vi "main.vi"() -> ()   [LabVIEW 2009, in "NavScreen.lvlib"]
uses:
  NavScreen.lvlib
  ItemIcon.ctl
  Classes/Link/Link.lvclass
  Classes/RingItem/RingItem.lvclass
panel:
  in  "stop":bool
  in  "Launch Project Wizard for Target":bool
  in  "Target Devices":u16(ring) items=["Real-Time Project"]
  in  "DNL_Column1Section3TopAlignment":bool caption="Find Examples..."
  in  "DNL_FileColumnLeftAlignment":string
  in  "DNL_ResourceColumnLeftAlignment":string
  in  "Ring 2-13":T1
  in  "Ring 2-14":T1
  in  "Ring 2-15":T1
  in  "Ring 2-16":T1
  in  "Ring 2-11":T1
  in  "Ring 2-10":T1
  in  "Ring 2-9":T1
  in  "Ring 2-8":T1
  in  "Ring 2-7":T1
  in  "Ring 2-6":T1
  in  "Ring 2-5":T1
  out "File":string="Column One"
  out "Resources":string="Column Two"
  in  "DNL_Link Button 25":bool caption="New To LabVIEW?"
  in  "DNL_Link Button 26":bool caption="Getting Started with LabVIEW"
  in  "DNL_Link Button 27":bool caption="LabVIEW Fundamentals"
  in  "DNL_Link Button 28":bool caption="Guide to LabVIEW Documentation"
  in  "DNL_Link Button 29":bool caption="LabVIEW Help"
  in  "DNL_Link Button 30":bool caption="Web Links"
  in  "DNL_Link Button 31":bool caption="Eyes on VIs (LabVIEW Blog)"
  in  "DNL_Link Button 32":bool caption="Darren's Weekly Nuggets"
  in  "DNL_Link Button 33":bool caption="LAVA"
  in  "DNL_Link Button 34":bool caption="LabVIEW Wiki"
  in  "DNL_Link Button 35":bool caption="More Web Resources"
  in  "DNL_Link Button 36":bool caption="Discussion Forums"
  in  "DNL_Link Button 37":bool caption="Training Courses"
  in  "DNL_Link Button 38":bool caption="LabVIEW Zone"
  in  "DNL_Link Button 39":bool caption="More Blogs"
  in  "DNL_Link Button 40":bool caption="NI Blog Listing"
  in  "DNL_Link Button 15":bool caption="Find Examples..."
  in  "DNL_Link Button 14":bool caption="Examples"
  in  "DNL_Link Button 13":bool caption="Browse..."
  in  "DNL_Link Button 12":bool caption="Untitled2.vi"
  in  "DNL_Link Button 11":bool caption="Targets"
  in  "DNL_Link Button 10":bool caption="Placeholder"
  in  "DNL_Link Button 9":bool caption="Placeholder"
  in  "DNL_Link Button 8":bool caption="Targets"
  in  "DNL_Link Button 7":bool caption="Browse..."
  in  "DNL_Link Button 6":bool caption="Section Header 2"
  in  "DNL_Link Button 5":bool caption="More..."
  in  "DNL_Link Button 4":bool caption="Placeholder"
  in  "DNL_Link Button 3":bool caption="Placeholder"
  in  "DNL_Link Button 2":bool caption="Real-Time Project"
  in  "DNL_Link Button 1":bool caption="Section Header"
  in  "DNL_Link Button 41":bool
  in  "DNL_Link Button 42":bool
  in  "DNL_Link Button 43":bool
  in  "DNL_Link Button 44":bool
  in  "DNL_Link Button 45":bool
  in  "DNL_Link Button 46":bool
  in  "DNL_Link Button 47":bool
  in  "DNL_Link Button 48":bool
  in  "DNL_Link Button 16":bool
  in  "DNL_Link Button 24":bool
  in  "DNL_Link Button 23":bool
  in  "DNL_Link Button 22":bool
  in  "DNL_Link Button 21":bool
  in  "DNL_Link Button 20":bool
  in  "DNL_Link Button 19":bool
  in  "DNL_Link Button 18":bool
  in  "DNL_Link Button 17":bool
  in  "Ring 2-4":T1
  in  "Ring 2-3":T1=1
  in  "Ring 2-2":T1=1
  in  "Ring 2":T1=8
  in  "Ring 2-12":T1
  out "Getting Started window":u16(ring)=2
  # "We size and scroll the panel programmatically during initialization. The background below is a picture ring.\n\nThe (off-screen) controls below define the left position of the two columns."
  # "This example demonstrates several aspects of LabVIEW object-oriented programming.\n\nIt is similar to the implementation of the LabVIEW Getting Started window.\n\nAn instance of a LabVIEW class handles each link on the dialog. Different classes handle different kinds of links (web URLs, help files, etc). All the classes inherit from Link.lvclass.\n\nThe private data of each class holds the information needed to perform the work of that class. For example, the Web.lvclass private data includes the URL to open.\n\nThe classes employ two kinds of dynamically dispatching member VIs. Some dynamic dispatching member VIs build upon the parent implementation of the VI, while others replace the parent implementation. The InitFromXML VIs extend the functionality of the parent classes by calling the parent implementation of the method and then doing additional work. The HandleItemActivation VIs override the parent class, substituting its work for whatever the parent class would have done in its absence.\n\nThe LinkItemFromXML.vi in Link.lvclass illustrates a \"factory\" design pattern.\n\nFinally, ProjectWizard.lvclass illustrates a helper class, allowing ProjectWizardClickableText.lvclass and RingItemProjectWizard.lvclass to share functionality without having a unique common ancestor class."
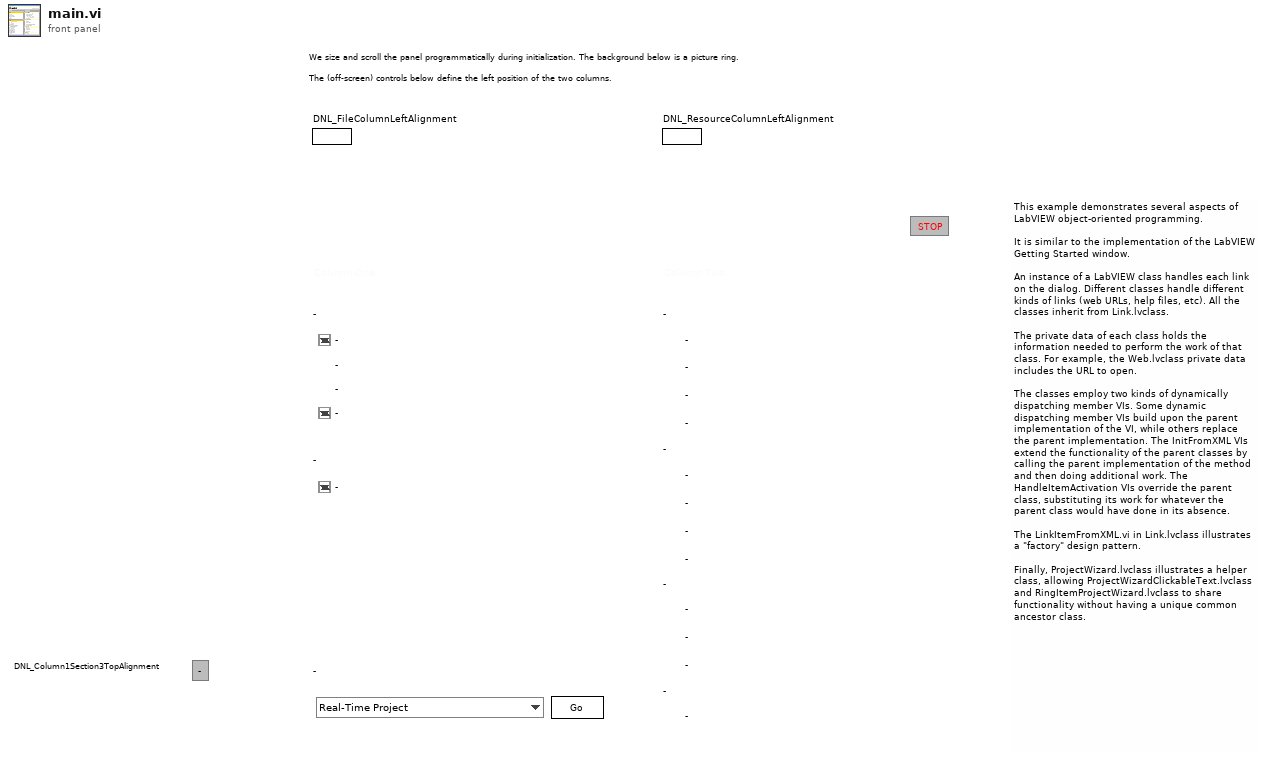
[diagram p1: front panel]
types:
  T1 = typedef "NavScreen.lvlib/ItemIcon.ctl" = u16
  T2 = cluster{refnum<class "ClickableText.lvclass">[]}[][]
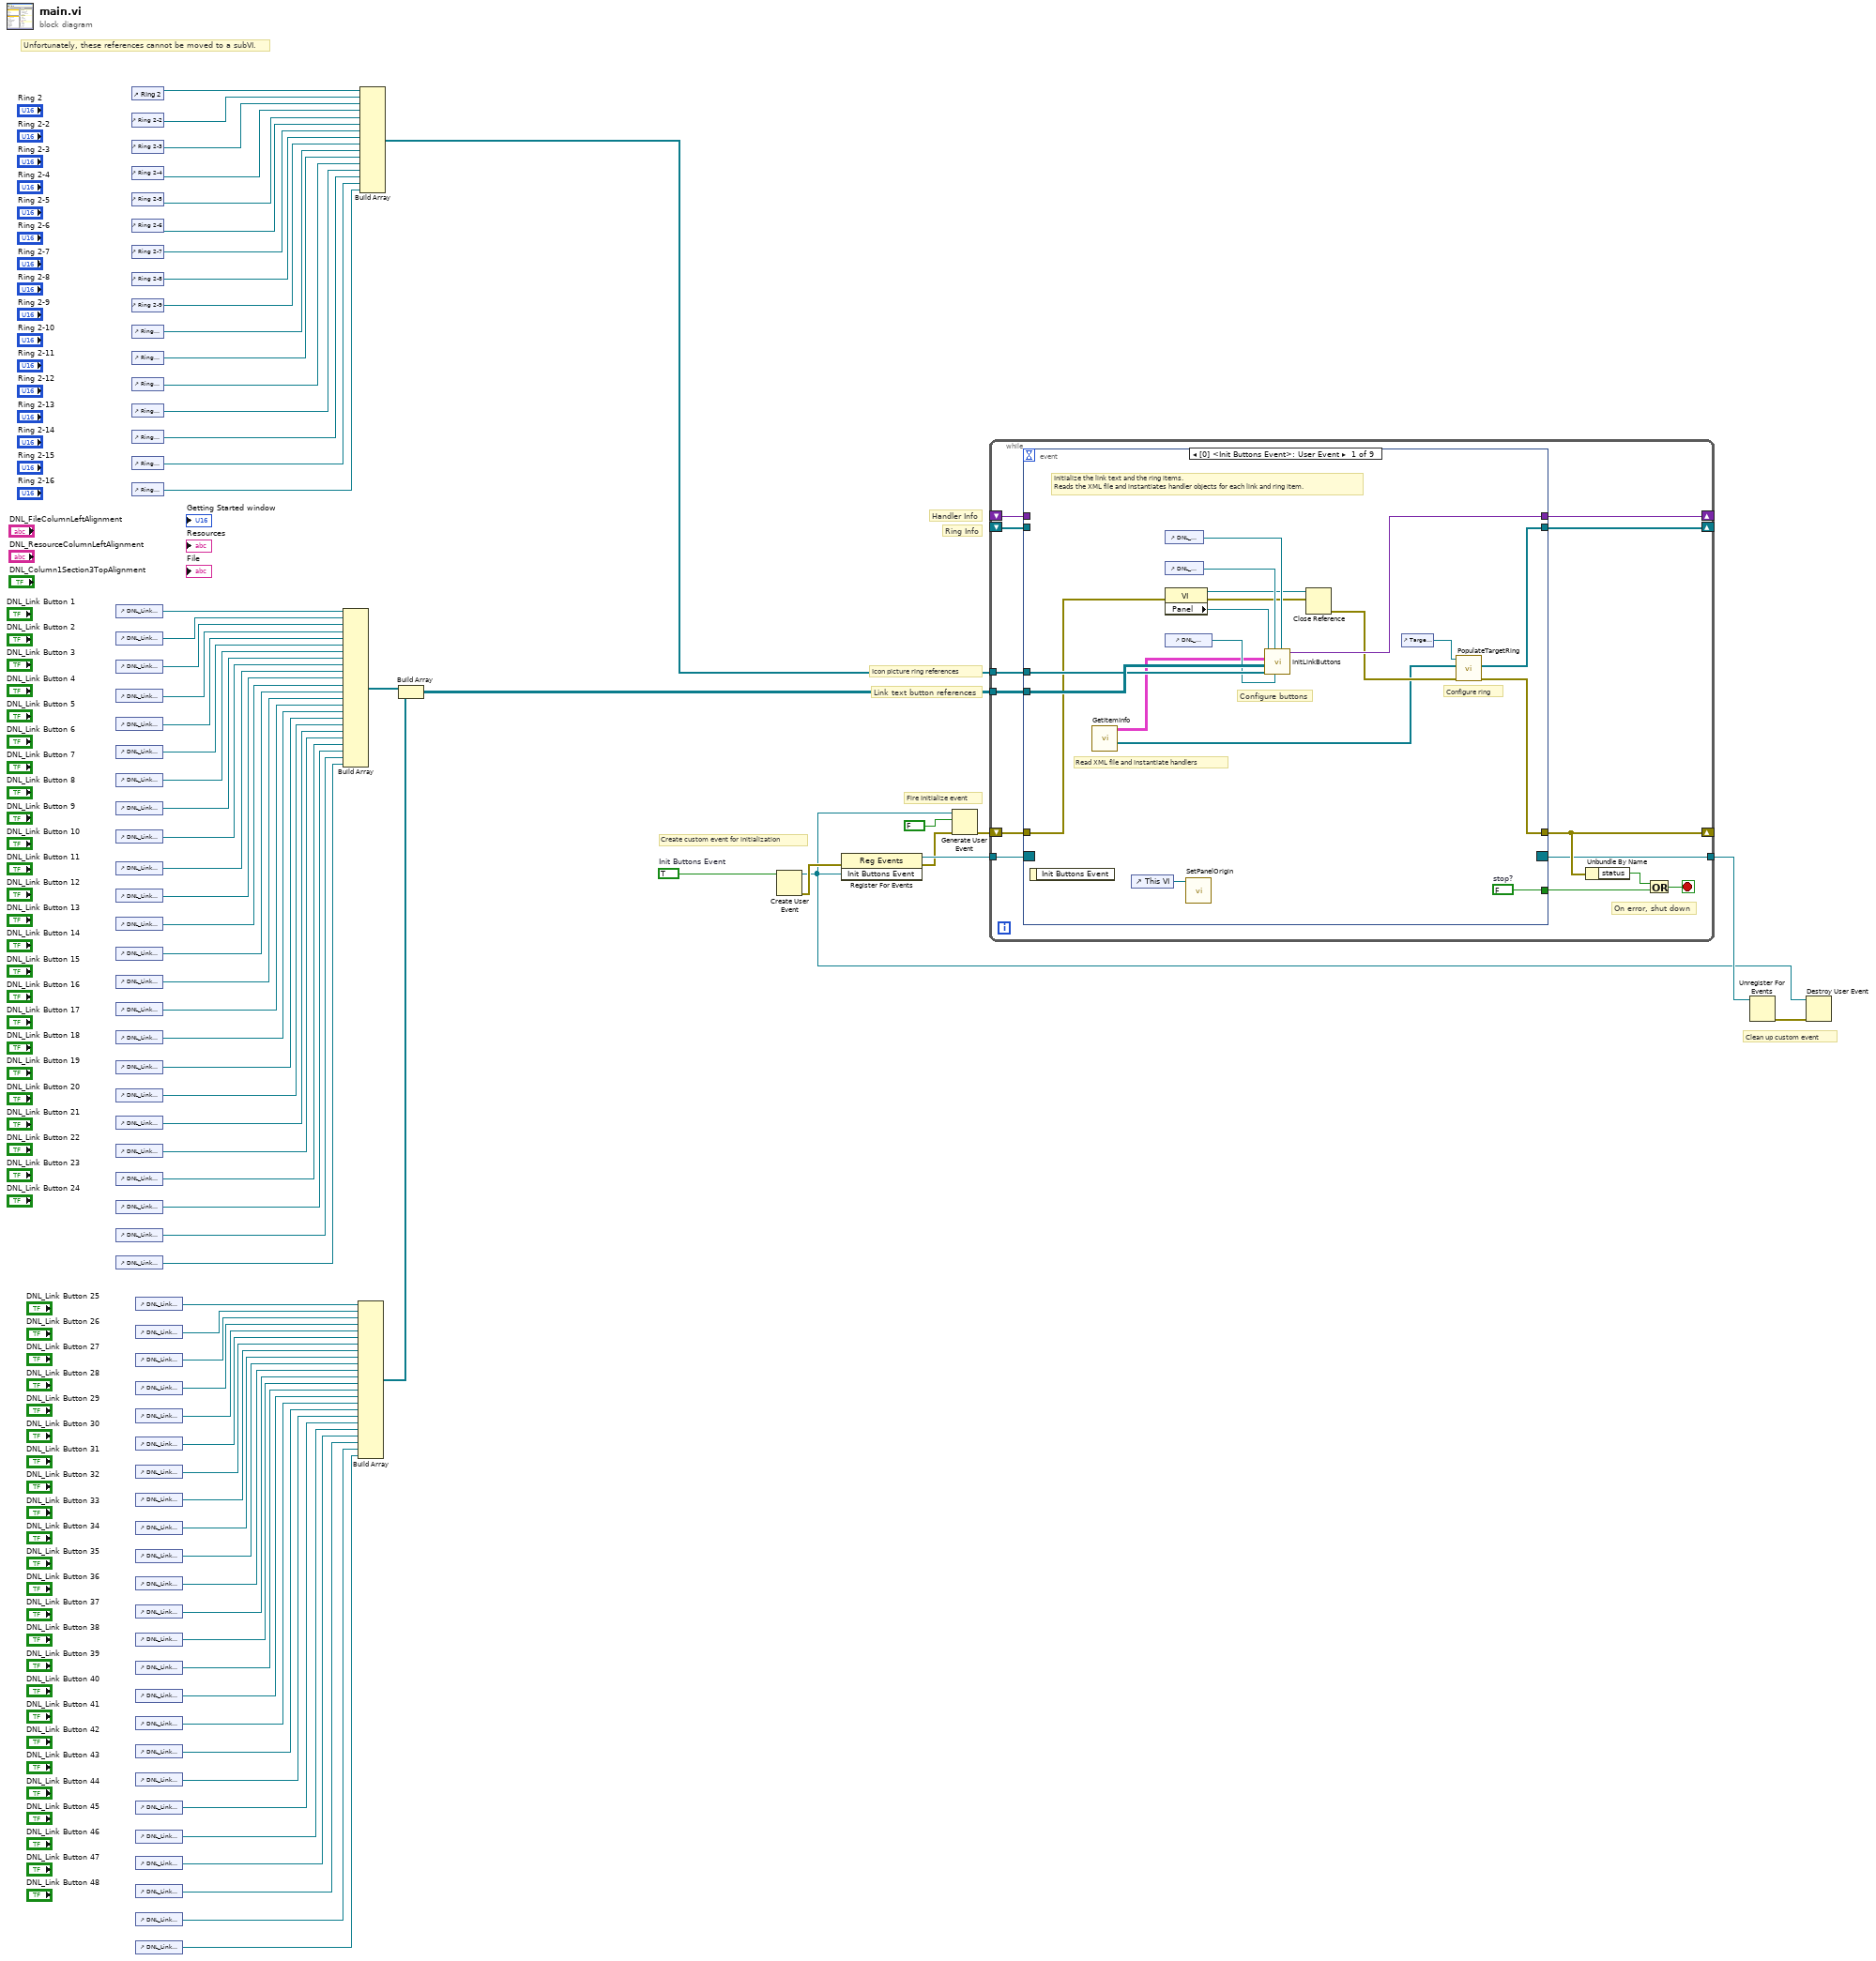
[diagram p0: block diagram]
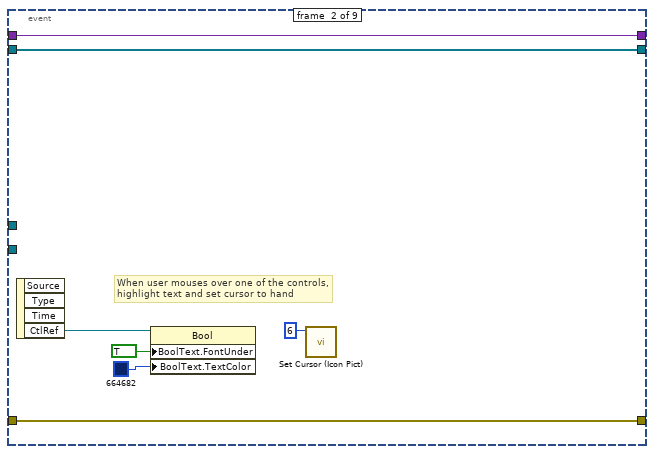
[diagram p2: hidden frame]
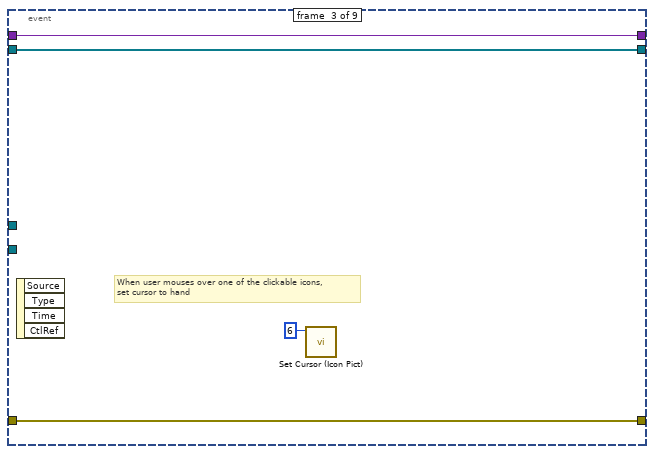
[diagram p3: hidden frame]
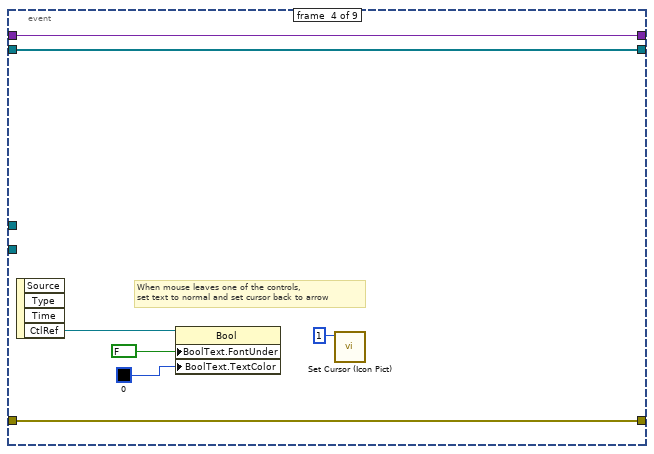
[diagram p4: hidden frame]
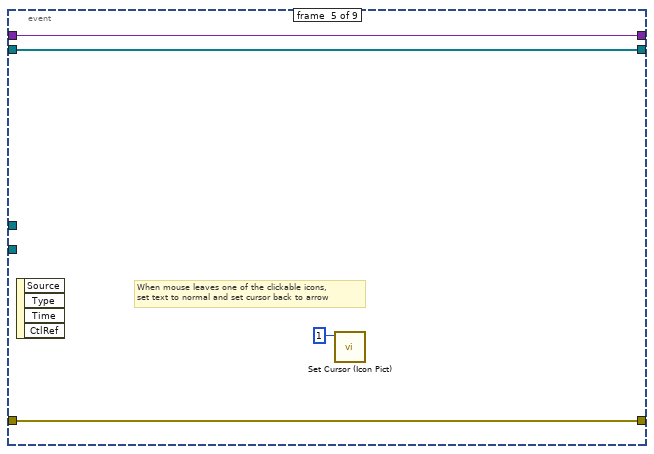
[diagram p5: hidden frame]
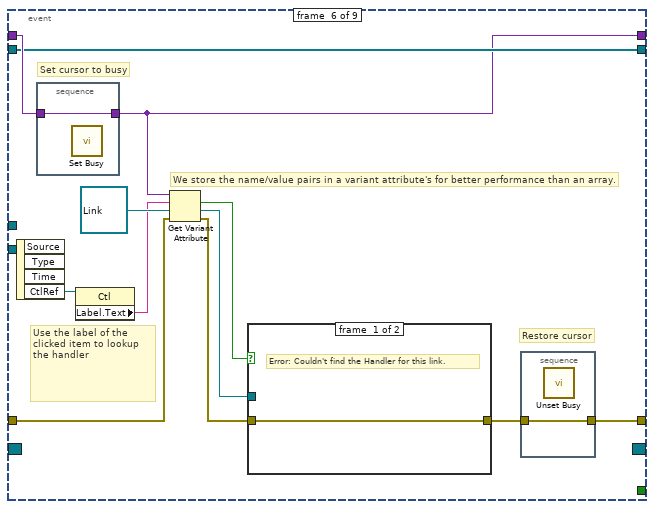
[diagram p6: hidden frame]
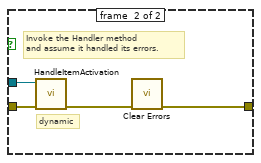
[diagram p7: hidden frame]
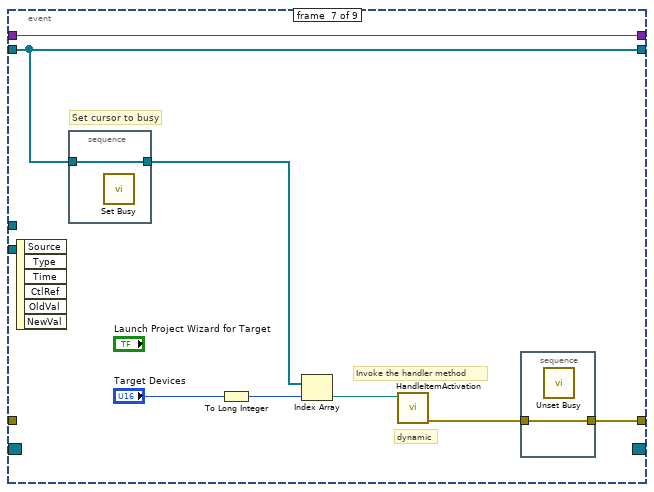
[diagram p8: hidden frame]
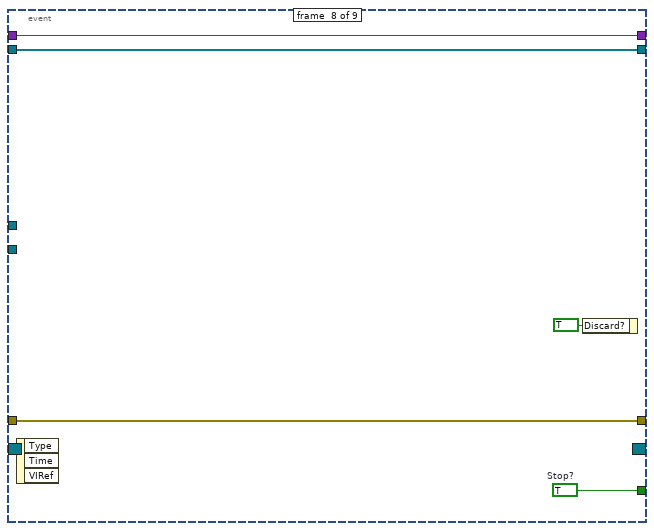
[diagram p9: hidden frame]
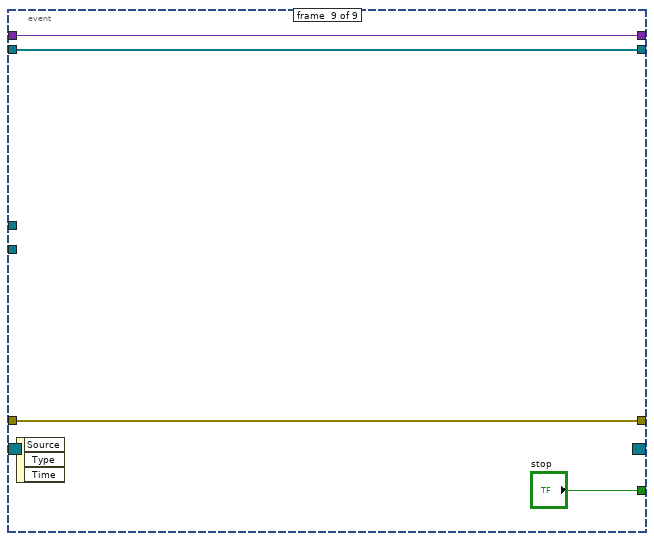
[diagram p10: hidden frame]
diagram:
  w5 = TRUE  # Init Buttons Event
  # "Unfortunately, these references cannot be moved to a subVI."
  # "Clean up custom event"
  # "Create custom event for initialization"
  # "Link text button references"
  # "Icon picture ring references"
  # "Ring Info"
  # "Handler Info"
  # "Fire Initialize event"
  n1 = control-ref of="DNL_Link Button 1"() -> (w77:refnum<vi>)
  n2 = control-ref of="DNL_Link Button 2"() -> (w76:refnum<vi>)
  n3 = control-ref of="DNL_Link Button 3"() -> (w75:refnum<vi>)
  n4 = control-ref of="DNL_Link Button 4"() -> (w74:refnum<vi>)
  n5 = control-ref of="DNL_Link Button 5"() -> (w73:refnum<vi>)
  n6 = control-ref of="DNL_Link Button 6"() -> (w72:refnum<vi>)
  n7 = control-ref of="DNL_Link Button 7"() -> (w71:refnum<vi>)
  n8 = control-ref of="DNL_Link Button 8"() -> (w70:refnum<vi>)
  n9 = control-ref of="DNL_Link Button 9"() -> (w69:refnum<vi>)
  n10 = control-ref of="DNL_Link Button 10"() -> (w68:refnum<vi>)
  n11 = control-ref of="DNL_Link Button 11"() -> (w67:refnum<vi>)
  n12 = control-ref of="DNL_Link Button 12"() -> (w54:refnum<vi>)
  n13 = control-ref of="DNL_Link Button 13"() -> (w66:refnum<vi>)
  n14 = control-ref of="DNL_Link Button 14"() -> (w65:refnum<vi>)
  n15 = control-ref of="DNL_Link Button 15"() -> (w64:refnum<vi>)
  n16 = control-ref of="DNL_Link Button 16"() -> (w63:refnum<vi>)
  n17 = control-ref of="DNL_Link Button 17"() -> (w62:refnum<vi>)
  n18 = control-ref of="DNL_Link Button 18"() -> (w61:refnum<vi>)
  n19 = control-ref of="DNL_Link Button 19"() -> (w60:refnum<vi>)
  n20 = control-ref of="DNL_Link Button 20"() -> (w59:refnum<vi>)
  n21 = control-ref of="DNL_Link Button 21"() -> (w58:refnum<vi>)
  n22 = control-ref of="DNL_Link Button 22"() -> (w57:refnum<vi>)
  n23 = control-ref of="DNL_Link Button 23"() -> (w56:refnum<vi>)
  n24 = control-ref of="DNL_Link Button 24"() -> (w55:refnum<vi>)
  n25 = control-ref of="Ring 2"() -> (w29:refnum<vi>)
  n26 = control-ref of="Ring 2-2"() -> (w28:refnum<vi>)
  n27 = control-ref of="Ring 2-3"() -> (w27:refnum<vi>)
  n28 = control-ref of="Ring 2-4"() -> (w26:refnum<vi>)
  n29 = control-ref of="Ring 2-5"() -> (w25:refnum<vi>)
  n30 = control-ref of="Ring 2-6"() -> (w24:refnum<vi>)
  n31 = control-ref of="Ring 2-7"() -> (w23:refnum<vi>)
  n32 = control-ref of="Ring 2-8"() -> (w22:refnum<vi>)
  n33 = control-ref of="Ring 2-9"() -> (w21:refnum<vi>)
  n34 = control-ref of="Ring 2-10"() -> (w20:refnum<vi>)
  n35 = control-ref of="Ring 2-11"() -> (w19:refnum<vi>)
  n36 = control-ref of="Ring 2-12"() -> (w18:refnum<vi>)
  n37 = control-ref of="Ring 2-13"() -> (w16:refnum<vi>)
  n38 = control-ref of="Ring 2-14"() -> (w15:refnum<vi>)
  n39 = control-ref of="Ring 2-15"() -> (w14:refnum<vi>)
  n40 = control-ref of="Ring 2-16"() -> (w13:refnum<vi>)
  n41 = control-ref of="DNL_Link Button 25"() -> (w53:refnum<vi>)
  n42 = control-ref of="DNL_Link Button 26"() -> (w52:refnum<vi>)
  n43 = control-ref of="DNL_Link Button 27"() -> (w51:refnum<vi>)
  n44 = control-ref of="DNL_Link Button 28"() -> (w50:refnum<vi>)
  n45 = control-ref of="DNL_Link Button 29"() -> (w49:refnum<vi>)
  n46 = control-ref of="DNL_Link Button 30"() -> (w48:refnum<vi>)
  n47 = control-ref of="DNL_Link Button 31"() -> (w47:refnum<vi>)
  n48 = control-ref of="DNL_Link Button 32"() -> (w46:refnum<vi>)
  n49 = control-ref of="DNL_Link Button 33"() -> (w45:refnum<vi>)
  n50 = control-ref of="DNL_Link Button 34"() -> (w44:refnum<vi>)
  n51 = control-ref of="DNL_Link Button 35"() -> (w43:refnum<vi>)
  n52 = control-ref of="DNL_Link Button 36"() -> (w42:refnum<vi>)
  n53 = control-ref of="DNL_Link Button 37"() -> (w41:refnum<vi>)
  n54 = control-ref of="DNL_Link Button 38"() -> (w40:refnum<vi>)
  n55 = control-ref of="DNL_Link Button 39"() -> (w39:refnum<vi>)
  n56 = control-ref of="DNL_Link Button 40"() -> (w38:refnum<vi>)
  n57 = control-ref of="DNL_Link Button 41"() -> (w37:refnum<vi>)
  n58 = control-ref of="DNL_Link Button 42"() -> (w36:refnum<vi>)
  n59 = control-ref of="DNL_Link Button 43"() -> (w35:refnum<vi>)
  n60 = control-ref of="DNL_Link Button 44"() -> (w34:refnum<vi>)
  n61 = control-ref of="DNL_Link Button 45"() -> (w33:refnum<vi>)
  n62 = control-ref of="DNL_Link Button 46"() -> (w32:refnum<vi>)
  n63 = control-ref of="DNL_Link Button 47"() -> (w31:refnum<vi>)
  n64 = control-ref of="DNL_Link Button 48"() -> (w30:refnum<vi>)
  n65 = Build Array(w77, w76, w75, w74, w73, w72, w71, w70, w69, w68, w67, w54, w66, w65, w64, w63, w62, w61, w60, w59, w58, w57, w56, w55) -> (w8:refnum<vi>[])
  n66 = Build Array(w53, w52, w51, w50, w49, w48, w47, w46, w45, w44, w43, w42, w41, w40, w39, w38, w37, w36, w35, w34, w33, w32, w31, w30) -> (w7:refnum<vi>[])
  n67 = Build Array(w29, w28, w27, w26, w25, w24, w23, w22, w21, w20, w19, w18, w16, w15, w14, w13) -> (w11:refnum<vi>[])
  n68 = Build Array(w8, w7) -> (w12:refnum<vi>[][])
  n69 = Create User Event(user event datatype=w5) -> (user event=w1:refnum<user-event>, error out=w6:errorcluster)  [unwired: 1 in]
  n70 = register-events(error in=w6, w1) -> (reference out=w17:refnum<event-registration>, error out=w4:errorcluster)  [unwired: 1 in]
  n71 = Generate User Event(user event=w1, event data cluster=FALSE ("event data"), error in=w4) -> (error out=w9:errorcluster)  [unwired: 1 out]
  n72 = while {
    shift-right: [w81] -> _
    shift-left: w9 -> [w83]
    tunnel: w17 -> [w89]
    shift-right: [w86] -> _
    shift-left: _ -> [w90]
    shift-right: [w84] -> _
    shift-left: _ -> [w85]
    tunnel: w12 -> [w88]
    tunnel: w11 -> [w87]
    tunnel: [w78] -> w3
    stop <- w79 stop-if-true
    # "On error, shut down"
    n73 = event shown="[0] <Init Buttons Event>: User Event" {
      selector: w89 -> [_ _ _ _ _ _ _ _ _]
      dyn-events: [_ _ _ _ _ _ _ _ _] -> w78
      timeout: _ -> [_ _ _ _ _ _ _ _ _]
      tunnel: [w102 _ _ _ _ _ _ w161 "stop"] -> w82
      tunnel: w90 -> [_ w111 w118 w122 w129 w141 w155 w163 w167]
      tunnel: [w104 w109 w116 w120 w127 w131 w157 w160 w165] -> w81
      tunnel: w88 -> [w108 _ _ _ _ _ _ _ _]
      tunnel: w87 -> [w107 _ _ _ _ _ _ _ _]
      tunnel: [w106 w111 w118 w122 w129 w138 w155 w163 w167] -> w86
      tunnel: w85 -> [_ w110 w117 w121 w128 w140 w154 w162 w166]
      tunnel: [w105 w110 w117 w121 w128 w140 w154 w162 w166] -> w84
      tunnel: w83 -> [w103 w109 w116 w120 w127 w136 _ w160 w165]
      event #0 {
        w102 = FALSE  # stop?
        # "Configure ring"
        # "Configure buttons"
        # "Read XML file and instantiate handlers"
        # "Initialize the link text and the ring items.\nReads the XML file and instantiates handler objects for each link and ring item."
        n74 = event-data() -> ()  [unwired: 1 in, 1 out]
        n75 = call "GetItemInfo.vi"() -> ("ring info"=w91:refnum<class "RingItem.lvclass">[], "item info array"=w92:T2)  [unwired: 10 in]
        n76 = control-ref of="This VI"() -> (w93:refnum<vi>)
        n77 = control-ref of="DNL_ResourceColumnLeftAlignment"() -> (w99:refnum<vi>)
        n78 = control-ref of="DNL_FileColumnLeftAlignment"() -> (w100:refnum<vi>)
        n79 = property on="Property Node" class="VI"(error in=w103) -> (reference out=w98:refnum<vi>, error out=w97:errorcluster, "Panel"=w101:refnum<vi>)  [unwired: 1 in]
        n80 = control-ref of="DNL_Column1Section3TopAlignment"() -> (w96:refnum<vi>)
        n81 = call "SetPanelOrigin.vi"("reference"=w93) -> ()  [unwired: 10 in, 1 out]
        n82 = call "InitLinkButtons.vi"("rightColumnAlignment"=w99, "Col1Sec3_Top"=w96, "leftColumnAlignment"=w100, "icon array"=w107, "button array"=w108, "item info array"=w92, "Pnl Refnum"=w101) -> ("Handler info"=w106:variant)  [unwired: 4 in]
        n83 = Close Reference(reference=w98, error in (no error)=w97) -> (error out=w94:errorcluster)
        n84 = control-ref of="Target Devices"() -> (w95:refnum<vi>)
        n85 = call "PopulateTargetRing.vi"("error in (no error)"=w94, "ring info"=w91, "Targets ring"=w95) -> ("error out"=w104:errorcluster, "ring info out"=w105:refnum<class "RingItem.lvclass">[])  [unwired: 7 in]
      }
      event #1 {
        # "When user mouses over one of the controls,\nhighlight text and set cursor to hand"
        n86 = event-data() -> ("CtlRef"=w115:refnum<vi>)  [unwired: 1 in, 3 out]
        n87 = property on="Property Node" class="Bool"(reference=w115, "BoolText.FontUnder"=TRUE ("Boolean Text.Font:Underline"), "BoolText.TextColor"=u32 664682) -> ()  [unwired: 1 in, 2 out]
        n88 = call <vilib>:"Set Cursor (Icon Pict).vi"("icon"=u16 6) -> ()  [unwired: 9 in, 2 out]
      }
      event #2 {
        # "When user mouses over one of the clickable icons,\nset cursor to hand"
        n89 = event-data() -> ()  [unwired: 1 in, 4 out]
        n90 = call <vilib>:"Set Cursor (Icon Pict).vi"("icon"=u16 6) -> ()  [unwired: 9 in, 2 out]
      }
      event #3 {
        # "When mouse leaves one of the controls,\nset text to normal and set cursor back to arrow"
        n91 = event-data() -> ("CtlRef"=w126:refnum<vi>)  [unwired: 1 in, 3 out]
        n92 = property on="Property Node" class="Bool"(reference=w126, "BoolText.FontUnder"=FALSE ("Boolean Text.Font:Underline"), "BoolText.TextColor"=u32 0) -> ()  [unwired: 1 in, 2 out]
        n93 = call <vilib>:"Set Cursor (Icon Pict).vi"("icon"=u16 1) -> ()  [unwired: 9 in, 2 out]
      }
      event #4 {
        # "When mouse leaves one of the clickable icons,\nset text to normal and set cursor back to arrow"
        n94 = event-data() -> ()  [unwired: 1 in, 4 out]
        n95 = call <vilib>:"Set Cursor (Icon Pict).vi"("icon"=u16 1) -> ()  [unwired: 9 in, 2 out]
      }
      event #5 {
        # "Use the label of the clicked item to lookup the handler"
        # "Restore cursor"
        # "We store the name/value pairs in a variant attribute's for better performance than an array."
        # "Set cursor to busy"
        n96 = event-data() -> ("CtlRef"=w142:refnum<vi>)  [unwired: 1 in, 3 out]
        n97 = stacked-sequence {
          tunnel: w141 -> [w144]
          tunnel: [w144] -> w138
          frame #0 {
            n98 = call <vilib>:"Set Busy.vi"() -> ()  [unwired: 10 in, 2 out]
          }
        }
        n99 = property on="Property Node" class="Ctl"(reference=w142) -> ("Label.Text"=w137:string)  [unwired: 1 in, 2 out]
        n100 = Get Variant Attribute(Variant=w138, name=w137, default value (empty Variant)=refnum<class "Link.lvclass"> refnum ("GettingStartedWindow.lvlib:Link.lvclass"), error in=w136) -> (found=w134:bool, value=w133:refnum<class "Link.lvclass">, error out=w135:errorcluster)  [unwired: 1 out]
        n101 = case shown="True" w134 {
          tunnel: [w145 w146] -> w132
          tunnel: w135 -> [w145 w149]
          tunnel: w133 -> [_ w148]
          frame #0 {
            # "Error: Couldn't find the Handler for this link."
          }
          frame #1 {
            # "dynamic"
            # "Invoke the Handler method\nand assume it handled its errors."
            n102 = call-dynamic "HandleItemActivation.vi"("error in (no error)"=w149, "Link in"=w148) -> ("error out"=w147:errorcluster)  [unwired: 8 in, 1 out]
            n103 = call <vilib>:"Clear Errors.vi"("error in (no error)"=w147) -> ("error out"=w146:errorcluster)  [unwired: 6 in]
          }
        }
        n104 = stacked-sequence {
          tunnel: [w143] -> w131
          tunnel: w132 -> [w143]
          frame #0 {
            n105 = call <vilib>:"Unset Busy.vi"() -> ()  [unwired: 11 in, 1 out]
          }
        }
      }
      event #6 {
        # "Invoke the handler method"
        # "dynamic"
        # "Set cursor to busy"
        n106 = event-data() -> ()  [unwired: 1 in, 6 out]
        n107 = stacked-sequence {
          tunnel: w154 -> [w159]
          tunnel: [w159] -> w153
          frame #0 {
            n108 = call <vilib>:"Set Busy.vi"() -> ()  [unwired: 10 in, 2 out]
          }
        }
        n109 = To Long Integer(number="Target Devices") -> (32bit integer=w151:i32)
        n110 = Index Array(array=w153, index=w151) -> (element=w152:refnum<class "RingItem.lvclass">)
        n111 = call-dynamic "HandleItemActivation.vi"("Link in"=w152) -> ("error out"=w150:errorcluster)  [unwired: 9 in, 1 out]
        n112 = stacked-sequence {
          tunnel: [w158] -> w157
          tunnel: w150 -> [w158]
          frame #0 {
            n113 = call <vilib>:"Unset Busy.vi"() -> ()  [unwired: 11 in, 1 out]
          }
        }
      }
      event #7 {
        w161 = TRUE  # Stop?
        n114 = event-data() -> ()  [unwired: 1 in, 3 out]
        n115 = event-data("Discard?"=TRUE) -> ()  [unwired: 1 in, 1 out]
      }
      event #8 {
        n116 = event-data() -> ()  [unwired: 1 in, 3 out]
      }
    }
    n117 = Unbundle By Name(w81) -> ("status"=w80:bool)
    n118 = Or(x=w80, y=w82) -> (x .or. y?=w79:bool)
  }
  n119 = Unregister For Events(event registration refnum=w3) -> (error out=w2:errorcluster)  [unwired: 1 in]
  n120 = Destroy User Event(user event=w1, error in=w2) -> ()  [unwired: 1 out]
